vi "Autonomous Independent.vi"() -> ()   [LabVIEW 2018]
doc: "This VI is called when autonomous begins, and will automatically be terminated when autonomous ends. You can carry out timed or sensor driven robot movement independently without needing to return to the caller."
uses:
  <vilib>/Rock Robotics/WPI/Utilities/WPI_GetSetVariantRefNum.vi
  <vilib>/Rock Robotics/Network Tables/NT Read String.vi
  <vilib>/Rock Robotics/Network Tables/NT Write Numeric Array.vi
  <vilib>/Rock Robotics/WPI/RobotDrive/WPI_RobotDriveArcadeDrive_Standard(NoSaturation).vi
panel:
  out "Current Movement, for debugging":T1 {"Y Joystick Value" scale=1.0..-1.0; "X Joystick Value" scale=-1.0..1.0}
  in  "Array of robot movements":T2(array[cluster])=[{"X Joystick Value"=0.39393939393939403, "Y Joystick Value"=0.0, "Delay (sec)"=1.0, "Movement Name"="turn"}, {"X Joystick Value"=-0.3737373737373737, "Y Joystick Value"=0.0, "Delay (sec)"=1.0, "Movement Name"="turn back"}] {"Y Joystick Value" scale=1.0..-1.0; "X Joystick Value" scale=-1.0..1.0}
  # "Be sure to right-click and choose Data Operations>>Make Current Value default if you want to save the array values with the VI"
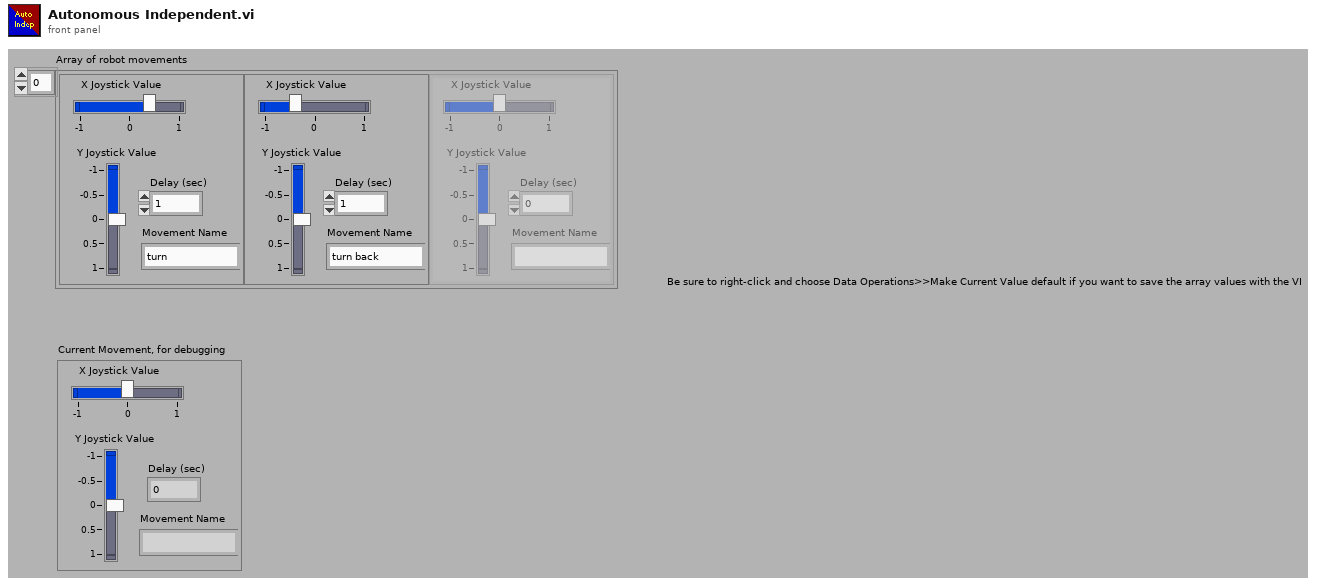
[diagram p1: front panel]
types:
  T1 = cluster{"X Joystick Value":dbl, "Y Joystick Value":dbl, "Delay (sec)":dbl, "Movement Name":string}
  T2 = cluster{"X Joystick Value":dbl, "Y Joystick Value":dbl, "Delay (sec)":dbl, "Movement Name":string}[]
  T3 = typedef "WPI_JoystickDevRef.ctl" = cluster{"Device":T4}
  T4 = typedef "WPI_JoystickDeviceEnum.ctl" = enum16{"USB 0", "USB 1", "USB 2", "USB 3", "USB 4", "USB 5"}
  T5 = typedef "WPI_RobotDriveDevRef.ctl" = cluster{"DevStatus":errorcluster, "Motors[]":T6[], "Square Inputs":bool, "Max Output":dbl}
  T6 = typedef "WPI_MotorControlDeviceRef.ctl" = cluster{"DeviceStatus":errorcluster, "Type":T7, "PWM":cluster{"PWM Channel":T8, "DeadBand":T9}, "CAN":cluster{"Device Number":u8, "SetOutput VI Ref":variant, "GetOutput VI Ref":variant, "Enable VI Ref":variant, "Disable VI Ref":variant, "Data":variant}, "Invert":bool, "DIO PWM":cluster{"PWM \"Enable\" Channel":T8, "DIOChannel":T10, "PWM Rate":dbl}}
  T7 = typedef "WPI_MotorControlType.ctl" = enum16{"PWM", "CAN", "DIO PWM"}
  T8 = typedef "FPGA_DIOPWMChannel.ctl" = enum8{"PWM 0", "PWM 1", "PWM 2", "PWM 3", "PWM 4", "PWM 5", "PWM 6", "PWM 7", "PWM 8", "PWM 9", "PWM MXP 0", "PWM MXP 1", "PWM MXP 2", "PWM MXP 3", "PWM MXP 4", "PWM MXP 5", "PWM MXP 6", "PWM MXP 7", "PWM MXP 8", "PWM MXP 9", "Invalid"}
  T9 = typedef "WPI_PWMDeadband.ctl" = cluster{"Name":string, "maxPositivePwm":i32, "minPositivePwm":i32, "centerPwm":i32, "maxNegativePwm":i32, "minNegativePwm":i32, "angularRange":u16}
  T10 = typedef "FPGA_DIOChannel.ctl" = enum8{"DIO 0", "DIO 1", "DIO 2", "DIO 3", "DIO 4", "DIO 5", "DIO 6", "DIO 7", "DIO 8", "DIO 9", "DIO MXP 0", "DIO MXP 1", "DIO MXP 2", "DIO MXP 3", "DIO MXP 4", "DIO MXP 5", "DIO MXP 6", "DIO MXP 7", "DIO MXP 8", "DIO MXP 9", "DIO MXP 10", "DIO MXP 11", "DIO MXP 12", "DIO MXP 13", "DIO MXP 14", "DIO MXP 15", "SPI Port CS1", "SPI Port CS2", "SPI Port CS3", "SPI Port MISO", "SPI Port MOSI", "Invalid"}
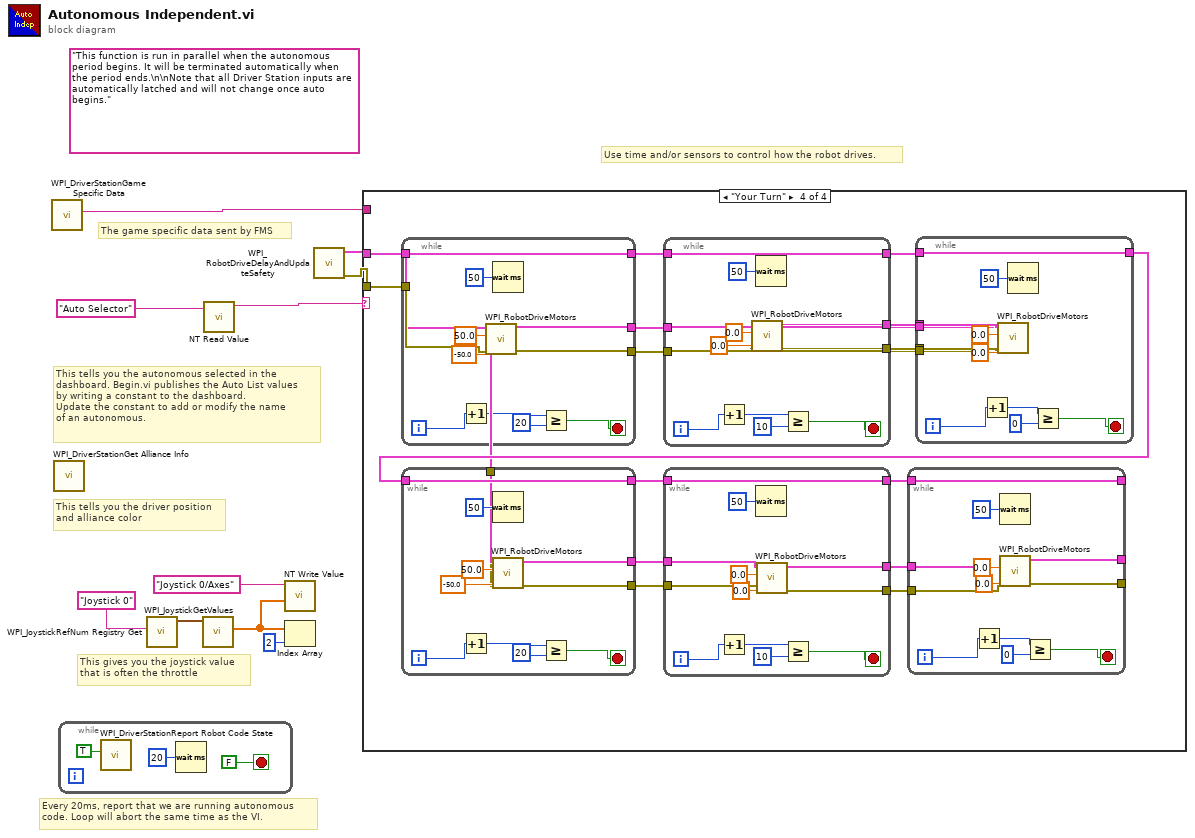
[diagram p0: block diagram]
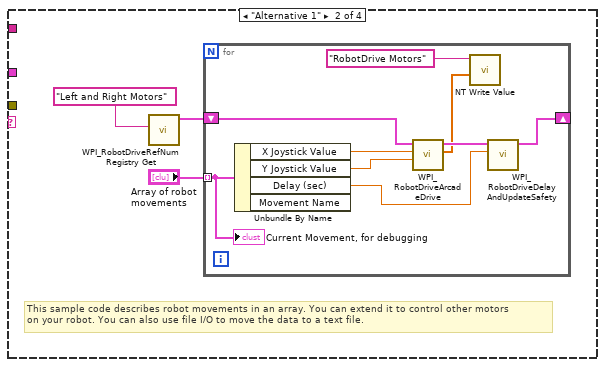
[diagram p3: hidden frame]
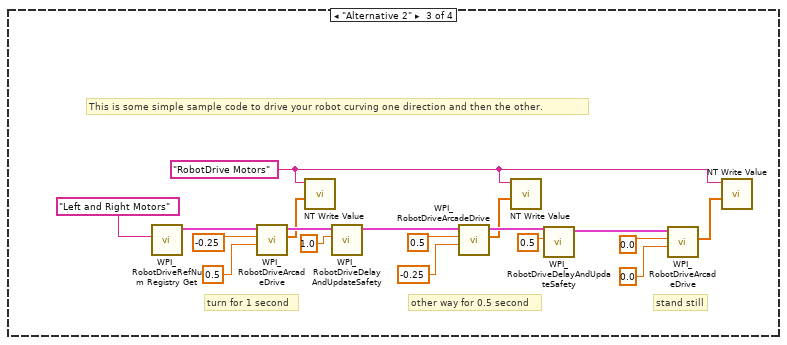
[diagram p4: hidden frame]
diagram:
  (unwired) "This function is run in parallel when the autonomous period begins. It will be terminated automatically when the period ends.\n\nNote that all Driver Station inputs are automatically latched and will not change once auto begins."
  # "The game specific data sent by FMS"
  # "This tells you the autonomous selected in the \ndashboard. Begin.vi publishes the Auto List values\nby writing a constant to the dashboard.\nUpdate the constant to add or modify the name\nof an autonomous."
  # "Every 20ms, report that we are running autonomous\ncode. Loop will abort the same time as the VI."
  # "This gives you the joystick value\nthat is often the throttle"
  # "This tells you the driver position\nand alliance color"
  # "Use time and/or sensors to control how the robot drives."
  n1 = call <vilib>:"WPI_DriverStationGame Specific Data.vi"() -> ("Game Specific Data"=w3:string)  [unwired: 11 in]
  n2 = call <vilib>:"WPI_DriverStationGet Alliance Info.vi"() -> ()  [unwired: 12 out]
  n3 = while {
    stop <- FALSE stop-if-true
    n4 = call <vilib>:"WPI_DriverStationReport Robot Code State.vi"("Autonomous"=TRUE) -> ()  [unwired: 10 in, 1 out]
    n5 = Wait (ms)(milliseconds to wait=u32 20) -> ()  [unwired: 1 out]
  }
  n6 = call <vilib>:"WPI_JoystickRefNum Registry Get.vi"("refnum name"="Joystick 0") -> ("JoystickDevRef"=w9:T3)  [unwired: 1 in, 9 out]
  n7 = call <vilib>:"WPI_JoystickGetValues.vi"("JoystickDevRef"=w9) -> ("Axes"=w5:dbl[])  [unwired: 6 in, 4 out]
  n8 = call-poly <vilib>:"NT Read Value.vi"("Name"="Auto Selector") -> ("String"=w6:string)  [unwired: 9 in, 1 out]
  n9 = call-poly <vilib>:"NT Write Value.vi"("Numeric Array"=w5, "Name"="Joystick 0/Axes") -> ()  [unwired: 9 in, 1 out]
  n10 = Index Array(array=w5, index=2) -> ()  [unwired: 1 out]
  n11 = call <vilib>:"WPI_RobotDriveDelayAndUpdateSafety.vi"() -> ("error out"=w1:errorcluster, "RobotDriveDevRef 2"=w2:T5)  [unwired: 10 in]
  n12 = case shown="\"Your Turn\"" w6 {
    tunnel: w3 -> [_ _ _ _]
    tunnel: w2 -> [_ _ _ w60]
    tunnel: w1 -> [_ _ _ w44]
    frame Default {
      # "You can put your main auto here, or you can right-click on the case and make any\nother frame be the default case."
      # "This is the frame that will execute if no selection is made, or if it is not recognized"
    }
    frame "Alternative 1" {
      # "This sample code describes robot movements in an array. You can extend it to control other motors\non your robot. You can also use file I/O to move the data to a text file."
      n13 = call <vilib>:"WPI_RobotDriveRefNum Registry Get.vi"("refnum name"="Left and Right Motors") -> ("RobotDriveDevRef"=w15:T5)  [unwired: 1 in, 9 out]
      n14 = for {
        shift-right: [w23] -> _
        shift-left: w15 -> [w24]
        tunnel: "Array of robot movements" -> [w19] mode=indexing
        n15 = Unbundle By Name(w19) -> ("X Joystick Value"=w22:dbl, "Y Joystick Value"=w21:dbl, "Delay (sec)"=w20:dbl)  [unwired: 1 out]
        n16 = call-poly <vilib>:"WPI_RobotDriveArcadeDrive.vi"("Y axis value"=w21, "X axis value"=w22, "RobotDriveDevRef"=w24) -> ("Motor Values"=w17:dbl[], "RobotDriveDevRef"=w25:T5)  [unwired: 1 in, 6 out]
        n17 = call-poly <vilib>:"NT Write Value.vi"("Numeric Array"=w17, "Name"="RobotDrive Motors") -> ()  [unwired: 9 in, 1 out]
        n18 = call <vilib>:"WPI_RobotDriveDelayAndUpdateSafety.vi"("Delay (s)"=w20, "RobotDriveDevRef"=w25) -> ("RobotDriveDevRef 2"=w23:T5)  [unwired: 8 in, 1 out]
        "Current Movement, for debugging" <- w19
      }
    }
    frame "Alternative 2" {
      w27 = "RobotDrive Motors" ("Name")
      # "This is some simple sample code to drive your robot curving one direction and then the other."
      # "stand still"
      # "other way for 0.5 second"
      # "turn for 1 second"
      n19 = call <vilib>:"WPI_RobotDriveRefNum Registry Get.vi"("refnum name"="Left and Right Motors") -> ("RobotDriveDevRef"=w43:T5)  [unwired: 1 in, 9 out]
      n20 = call-poly <vilib>:"WPI_RobotDriveArcadeDrive.vi"("Y axis value"=0.5 ("X axis value"), "X axis value"=-0.25, "RobotDriveDevRef"=w43) -> ("Motor Values"=w26:dbl[], "RobotDriveDevRef"=w36:T5)  [unwired: 1 in, 6 out]
      n21 = call-poly <vilib>:"NT Write Value.vi"("Numeric Array"=w26, "Name"=w27) -> ()  [unwired: 9 in, 1 out]
      n22 = call <vilib>:"WPI_RobotDriveDelayAndUpdateSafety.vi"("Delay (s)"=1.0, "RobotDriveDevRef"=w36) -> ("RobotDriveDevRef 2"=w37:T5)  [unwired: 8 in, 1 out]
      n23 = call-poly <vilib>:"WPI_RobotDriveArcadeDrive.vi"("Y axis value"=-0.25 ("X axis value"), "X axis value"=0.5, "RobotDriveDevRef"=w37) -> ("Motor Values"=w28:dbl[], "RobotDriveDevRef"=w38:T5)  [unwired: 1 in, 6 out]
      n24 = call-poly <vilib>:"NT Write Value.vi"("Numeric Array"=w28, "Name"=w27) -> ()  [unwired: 9 in, 1 out]
      n25 = call <vilib>:"WPI_RobotDriveDelayAndUpdateSafety.vi"("Delay (s)"=0.5, "RobotDriveDevRef"=w38) -> ("RobotDriveDevRef 2"=w39:T5)  [unwired: 8 in, 1 out]
      n26 = call-poly <vilib>:"WPI_RobotDriveArcadeDrive.vi"("Y axis value"=0.0 ("X axis value"), "X axis value"=0.0, "RobotDriveDevRef"=w39) -> ("Motor Values"=w29:dbl[])  [unwired: 1 in, 7 out]
      n27 = call-poly <vilib>:"NT Write Value.vi"("Numeric Array"=w29, "Name"=w27) -> ()  [unwired: 9 in, 1 out]
    }
    frame "Your Turn" {
      n28 = while {
        tunnel: [w121] -> w59
        tunnel: w60 -> [w121]
        tunnel: [w124] -> w54
        tunnel: [w123] -> w53
        tunnel: w44 -> [w122]
        i -> [w131]
        stop <- w128 stop-if-true
        n29 = Increment(x=w131) -> (x+1=w130:i32)
        n30 = call <vilib>:"WPI_RobotDriveMotors.vi"("error in (no error)"=w122, "RightSpeed"=-50.0, "LeftSpeed"=50.0, "RobotDriveDevRef"=w121) -> ("error out"=w124:errorcluster, "RobotDriveDevRef"=w123:T5)  [unwired: 5 in, 1 out]
        n31 = Wait (ms)(milliseconds to wait=u32 50) -> ()  [unwired: 1 out]
        n32 = Greater Or Equal?(x=w130, y=20) -> (x >= y?=w128:bool)
      }
      n33 = while {
        tunnel: [w115] -> w58
        tunnel: w59 -> [w115]
        tunnel: w54 -> [w112]
        tunnel: w53 -> [w111]
        tunnel: [w110] -> w52
        tunnel: [w109] -> w51
        i -> [w118]
        stop <- w119 stop-if-true
        n34 = Increment(x=w118) -> (x+1=w117:i32)
        n35 = call <vilib>:"WPI_RobotDriveMotors.vi"("error in (no error)"=w112, "RightSpeed"=0.0, "LeftSpeed"=0.0, "RobotDriveDevRef"=w111) -> ("error out"=w109:errorcluster, "RobotDriveDevRef"=w110:T5)  [unwired: 5 in, 1 out]
        n36 = Wait (ms)(milliseconds to wait=u32 50) -> ()  [unwired: 1 out]
        n37 = Greater Or Equal?(x=w117, y=10) -> (x >= y?=w119:bool)
      }
      n38 = while {
        tunnel: [w103] -> w57
        tunnel: w58 -> [w103]
        tunnel: w52 -> [w100]
        tunnel: w51 -> [w99]
        tunnel: [w98] -> w50
        tunnel: [w97] -> w49
        i -> [w108]
        stop <- w106 stop-if-true
        n39 = Increment(x=w108) -> (x+1=w107:i32)
        n40 = call <vilib>:"WPI_RobotDriveMotors.vi"("error in (no error)"=w99, "RightSpeed"=0.0, "LeftSpeed"=0.0, "RobotDriveDevRef"=w100) -> ("error out"=w97:errorcluster, "RobotDriveDevRef"=w98:T5)  [unwired: 5 in, 1 out]
        n41 = Wait (ms)(milliseconds to wait=u32 50) -> ()  [unwired: 1 out]
        n42 = Greater Or Equal?(x=w107, y=0) -> (x >= y?=w106:bool)
      }
      n43 = while {
        tunnel: w57 -> [w92]
        tunnel: [w92] -> w56
        tunnel: w50 -> [w88]
        tunnel: w49 -> [w87]
        tunnel: [w86] -> w48
        tunnel: [w85] -> w47
        i -> [w96]
        stop <- w91 stop-if-true
        n44 = Increment(x=w96) -> (x+1=w95:i32)
        n45 = Wait (ms)(milliseconds to wait=u32 50) -> ()  [unwired: 1 out]
        n46 = call <vilib>:"WPI_RobotDriveMotors.vi"("error in (no error)"=w87, "RightSpeed"=-50.0, "LeftSpeed"=50.0, "RobotDriveDevRef"=w88) -> ("error out"=w85:errorcluster, "RobotDriveDevRef"=w86:T5)  [unwired: 5 in, 1 out]
        n47 = Greater Or Equal?(x=w95, y=20) -> (x >= y?=w91:bool)
      }
      n48 = while {
        tunnel: [w79] -> w55
        tunnel: w56 -> [w79]
        tunnel: w48 -> [w76]
        tunnel: w47 -> [w75]
        tunnel: [w74] -> w46
        tunnel: [w73] -> w45
        i -> [w82]
        stop <- w83 stop-if-true
        n49 = Increment(x=w82) -> (x+1=w81:i32)
        n50 = Wait (ms)(milliseconds to wait=u32 50) -> ()  [unwired: 1 out]
        n51 = call <vilib>:"WPI_RobotDriveMotors.vi"("error in (no error)"=w75, "RightSpeed"=0.0, "LeftSpeed"=0.0, "RobotDriveDevRef"=w76) -> ("error out"=w73:errorcluster, "RobotDriveDevRef"=w74:T5)  [unwired: 5 in, 1 out]
        n52 = Greater Or Equal?(x=w81, y=10) -> (x >= y?=w83:bool)
      }
      n53 = while {
        tunnel: [w67] -> _
        tunnel: w55 -> [w67]
        tunnel: w46 -> [w64]
        tunnel: w45 -> [w63]
        tunnel: [w62] -> _
        tunnel: [w61] -> _
        i -> [w72]
        stop <- w70 stop-if-true
        n54 = Increment(x=w72) -> (x+1=w71:i32)
        n55 = Wait (ms)(milliseconds to wait=u32 50) -> ()  [unwired: 1 out]
        n56 = call <vilib>:"WPI_RobotDriveMotors.vi"("error in (no error)"=w63, "RightSpeed"=0.0, "LeftSpeed"=0.0, "RobotDriveDevRef"=w64) -> ("error out"=w61:errorcluster, "RobotDriveDevRef"=w62:T5)  [unwired: 5 in, 1 out]
        n57 = Greater Or Equal?(x=w71, y=0) -> (x >= y?=w70:bool)
      }
    }
  }
